vi "Top Level.vi"() -> ()   [LabVIEW 2015]
uses:
  Brower Console/Controllers/Brower/BrowerController.lvclass
  File IO/Controllers/ProjectController/ProjectController.lvclass
  File IO/Controllers/Messages/Set BrowerController Ref_Msg/Set BrowerController Ref_Msg.lvclass/Set BrowerController Ref_Msg.ctl
  <vilib>/ActorFramework/Message Enqueuer/Message Enqueuer.lvclass/Message Enqueuer.ctl
  Brower Console/Controllers/Messages/Set ProjectController Ref_Msg/Set ProjectController Ref_Msg.lvclass/Set ProjectController Ref_Msg.ctl
  <vilib>/ActorFramework/Stop Msg/Stop Msg.lvclass/Stop Msg.ctl
  <vilib>/ActorFramework/Message Enqueuer/Enqueue.vi
  <vilib>/ActorFramework/Message Enqueuer/Enqueue Critical.vi
  <vilib>/ActorFramework/Message Priority Queue/Priority Enqueue.vi
  Brower Console/Controllers/Messages/Set ProjectController Ref_Msg/Set ProjectController Ref_Msg.lvclass
  File IO/Controllers/Messages/Set BrowerController Ref_Msg/Set BrowerController Ref_Msg.lvclass
  <vilib>/ActorFramework/Stop Msg/Stop Msg.lvclass
  <vilib>/ActorFramework/Actor/Actor.lvclass
panel:
  in  "Stop Button":bool
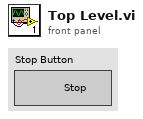
[diagram p1: front panel]
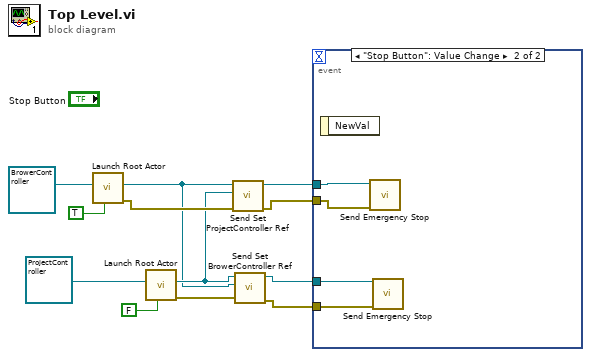
[diagram p0: block diagram]
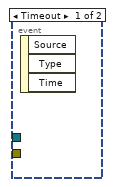
[diagram p2: hidden frame]
diagram:
  n1 = call <vilib>:"Launch Root Actor.vi"("Open Actor Core front panel? (F)"=TRUE, "Actor"=refnum<class "BrowerController.lvclass"> refnum ("BrowerController.lvclass")) -> ("error out"=w8:errorcluster, "Actor's Enqueuer"=w3:refnum<class "Message Enqueuer.lvclass">)  [unwired: 8 in]
  n2 = call <vilib>:"Launch Root Actor.vi"("Open Actor Core front panel? (F)"=FALSE, "Actor"=refnum<class "ProjectController.lvclass"> refnum ("ProjectController.lvclass")) -> ("error out"=w5:errorcluster, "Actor's Enqueuer"=w4:refnum<class "Message Enqueuer.lvclass">)  [unwired: 8 in]
  n3 = call "Send Set ProjectController Ref.vi"("error in (no error)"=w8, "ProjectController Ref"=w4, "Message Enqueuer"=w3) -> ("error out"=w6:errorcluster, "Message Enqueuer out"=w7:refnum<class "Message Enqueuer.lvclass">)  [unwired: 7 in]
  n4 = call "Send Set BrowerController Ref.vi"("error in (no error)"=w5, "BrowerController Ref"=w3, "Message Enqueuer"=w4) -> ("error out"=w1:errorcluster, "Message Enqueuer out"=w2:refnum<class "Message Enqueuer.lvclass">)  [unwired: 7 in]
  n5 = event shown="[1] \"Stop Button\": Value Change" {
    selector: _ -> [_ _]
    dyn-events: _ -> [_ _]
    timeout: _ -> [_ _]
    tunnel: w7 -> [_ w17]
    tunnel: w6 -> [w13 w14]
    tunnel: [w13 _] -> _
    tunnel: w2 -> [_ w16]
    tunnel: w1 -> [_ w15]
    event Timeout {
      n6 = event-data() -> ()  [unwired: 1 in, 3 out]
    }
    event "Stop Button": Value Change {
      n7 = event-data() -> ()  [unwired: 1 in, 1 out]
      n8 = call <vilib>:"Send Emergency Stop.vi"("error in (no error)"=w14, "Message Enqueuer"=w17) -> ()  [unwired: 9 in, 1 out]
      n9 = call <vilib>:"Send Emergency Stop.vi"("error in (no error)"=w15, "Message Enqueuer"=w16) -> ()  [unwired: 9 in, 1 out]
    }
  }
